vi "SEA_9811_Read_word.vi"(8 "error in (no error)":errorcluster, 9 "i":i32, 10 "channel #":u32, 11 "SEA9811_RT_data in":T1 {"Tx"."Tx Refs (Data,Trig)"."Data Reference" format="%.0x"}) -> (0 "error out":errorcluster, 1 "word":u32, 2 "SDI":u8, 3 "SEA9811_RT_data out":T1 {"Tx"."Tx Refs (Data,Trig)"."Data Reference" format="%.0x"}, 4 "timestamp":dbl, 5 "label":u8)   [LabVIEW 2015]
doc: "get label, SDI, word and timestamp for word[i] in channel[#]"
uses:
  Typdefs/SEA9811_RT_data_cluster.ctl
  <userlib>/_FPGA Interface Advanced Tools/FPGA Interface Base/FPGA Interface Base.lvclass
  Typdefs/FPGA ref.ctl
  Typdefs/channel.ctl
  Typdefs/received word.ctl
  Typdefs/SEA9811_FPGA_FP_Addresses.ctl
  <vilib>/NI Veristand/Custom Device API/Block Data Reference.ctl
  <vilib>/NI Veristand/Custom Device API/Data Reference.ctl
  <vilib>/NI VeriStand/Custom Device API/Custom Device API.lvlib
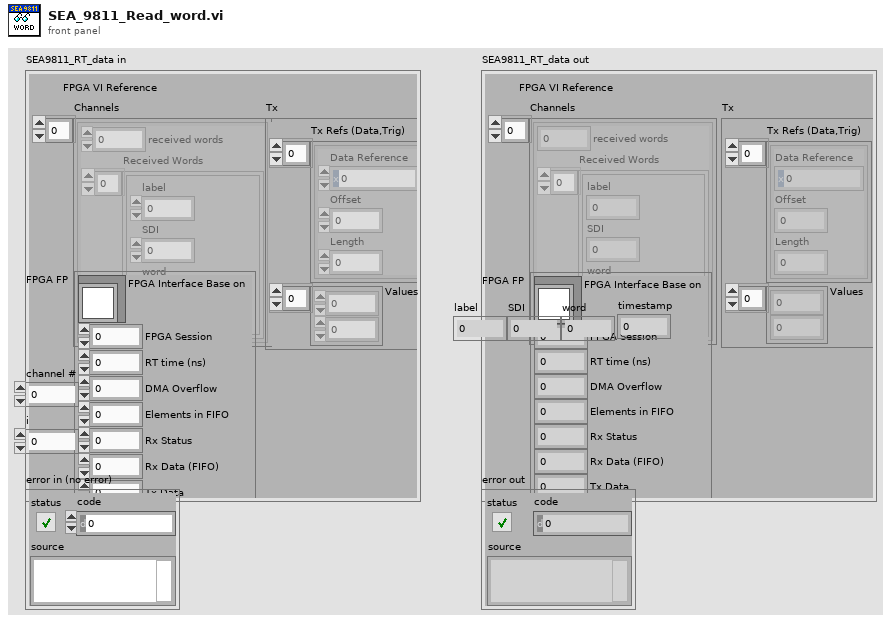
[diagram p1: front panel]
types:
  T1 = typedef "SEA9811_RT_data_cluster.ctl" = cluster{"FPGA VI Reference":T2, "Channels":T3[], "FPGA FP":T5, "Tx":cluster{"Tx Refs (Data,Trig)":T6[], "Values":dbl[]}}
  T2 = typedef "FPGA ref.ctl" = refnum<k20>
  T3 = typedef "channel.ctl" = cluster{"received words":u32, "Received Words":T4[]}
  T4 = typedef "received word.ctl" = cluster{"label":u8, "SDI":u8, "word":u32, "timestamp":dbl}
  T5 = typedef "SEA9811_FPGA_FP_Addresses.ctl" = cluster{"FPGA Interface Base on":refnum<class "FPGA Interface Base.lvclass">, "FPGA Session":u32, "RT time (ns)":u32, "DMA Overflow":u32, "Elements in FIFO":u32, "Rx Status":u32, "Rx Data (FIFO)":u32, "Tx Data":u32, "Transmit Data":u32}
  T6 = typedef "Custom Device API.lvlib/Block Data Reference.ctl" = cluster{"Data Reference":T7, "Offset":u64, "Length":u64}
  T7 = typedef "Custom Device API.lvlib/Data Reference.ctl" = i32
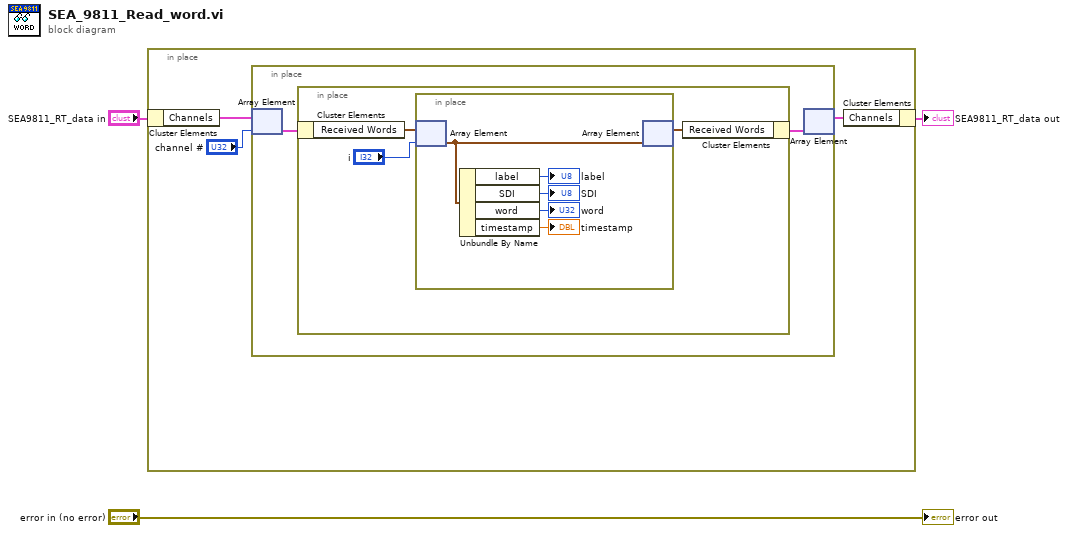
[diagram p0: block diagram]
diagram:
  n1 = in-place {
    n2 = in-place-cluster #1("SEA9811_RT_data in") -> ("Channels"=w6:T3[])
    n3 = in-place {
      n4 = in-place-array #2(w6, "channel #") -> (w8:T3)
      n5 = in-place {
        n6 = in-place-cluster #3(w8) -> ("Received Words"=w11:T4[])
        n7 = in-place {
          n8 = in-place-array #4(w11, "i") -> (w16:T4)
          n9 = Unbundle By Name(w16) -> ("label"=→"label":u8, "SDI"=→"SDI":u8, "word"=→"word":u32, "timestamp"=→"timestamp":dbl)
          n10 = in-place-array #4(w16) -> (w9:T4[])  [unwired: 1 out]
        }
        n11 = in-place-cluster #3("Received Words"=w9) -> (w7:T3)
      }
      n12 = in-place-array #2(w7) -> (w4:T3[])  [unwired: 1 out]
    }
    n13 = in-place-cluster #1("Channels"=w4) -> (→"SEA9811_RT_data out":T1)
  }
  "error out" <- "error in (no error)"
